vi "Read Digital In By Name.vi"(8 "error in":errorcluster, 10 "Name":string, 11 "DIG_IO in":refnum<class "DIG_IO.lvclass">) -> (0 "error out":errorcluster, 2 "State":bool, 3 "DIG_IO out":refnum<class "DIG_IO.lvclass">)   [LabVIEW 2019, in "DIG_IO.lvlib" / "DIG_IO.lvclass"]
uses:
  Library/DIG_IO.lvclass
  Library/DIG_IO.lvclass/DIG_IO.ctl
  Accessors/Read Channel Names.vi
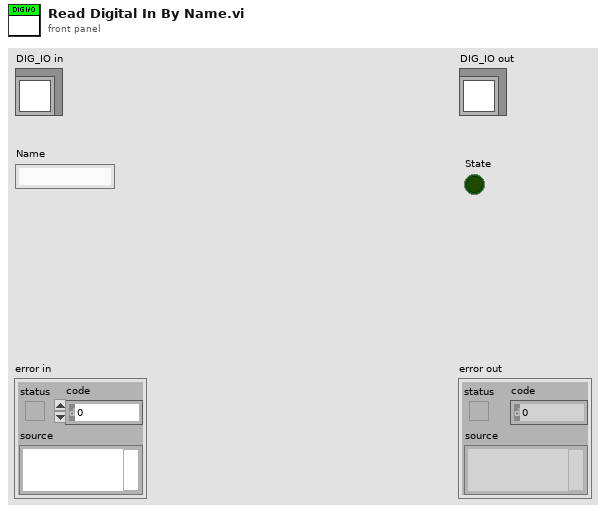
[diagram p1: front panel]
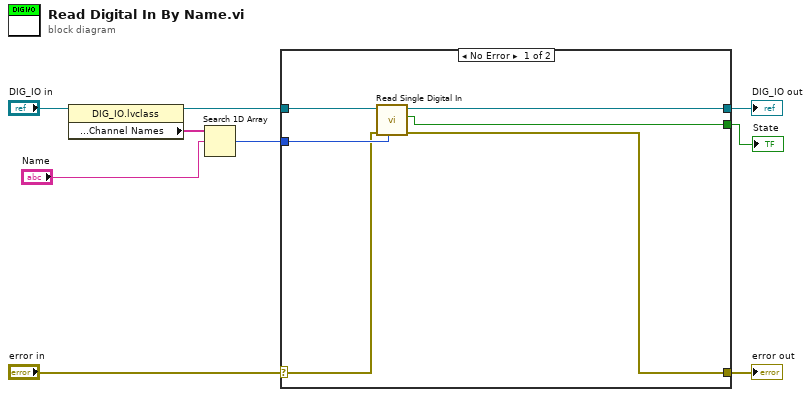
[diagram p0: block diagram]
diagram:
  n1 = property class="DIG_IO.lvclass"(reference="DIG_IO in") -> (reference out=w5:refnum<class "DIG_IO.lvclass">, "Accessors:Channel:Channel Names"=w4:string[])  [unwired: 1 in, 1 out]
  n2 = Search 1D Array(1D array=w4, element="Name") -> (index of element=w2:i32)  [unwired: 1 in]
  n3 = case shown="No Error" "error in" {
    selector: "error in" -> [w12 w17]
    tunnel: [w11 w17] -> w8
    tunnel: [w14 w16] -> w7
    tunnel: w5 -> [w15 w16]
    tunnel: w2 -> [w13 _]
    tunnel: [w10 _] -> w1
    frame No Error {
      n4 = call "Read Single Digital In.vi"("Value to Read"=w13, "error in"=w12, "DIG_IO in"=w15) -> ("error out"=w11:errorcluster, "Value"=w10:bool, "DIG_IO out"=w14:refnum<class "DIG_IO.lvclass">)  [unwired: 6 in]
    }
    frame Error {
    }
  }
  "error out" <- w8
  "DIG_IO out" <- w7
  "State" <- w1
